vi "Channel Probe_Find Specific VI.vi"(11 "element in":T1) -> (0 "error out":errorcluster, 2 "VI Refnum":refnum<vi>, 3 "element in":T1)   [LabVIEW 2019, in "MessengerM.lvlib"]
uses:
  MessengerM.lvlib
  <vilib>/ChannelSupport/Channel Message/Channel Message.lvclass
  Element.ctl
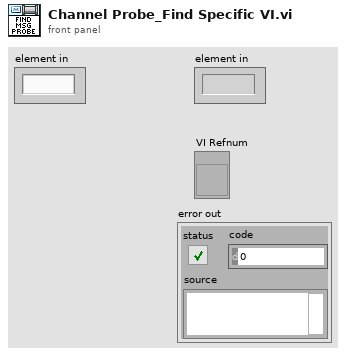
[diagram p1: front panel]
types:
  T1 = typedef "MessengerM.lvlib/Element.ctl" = string
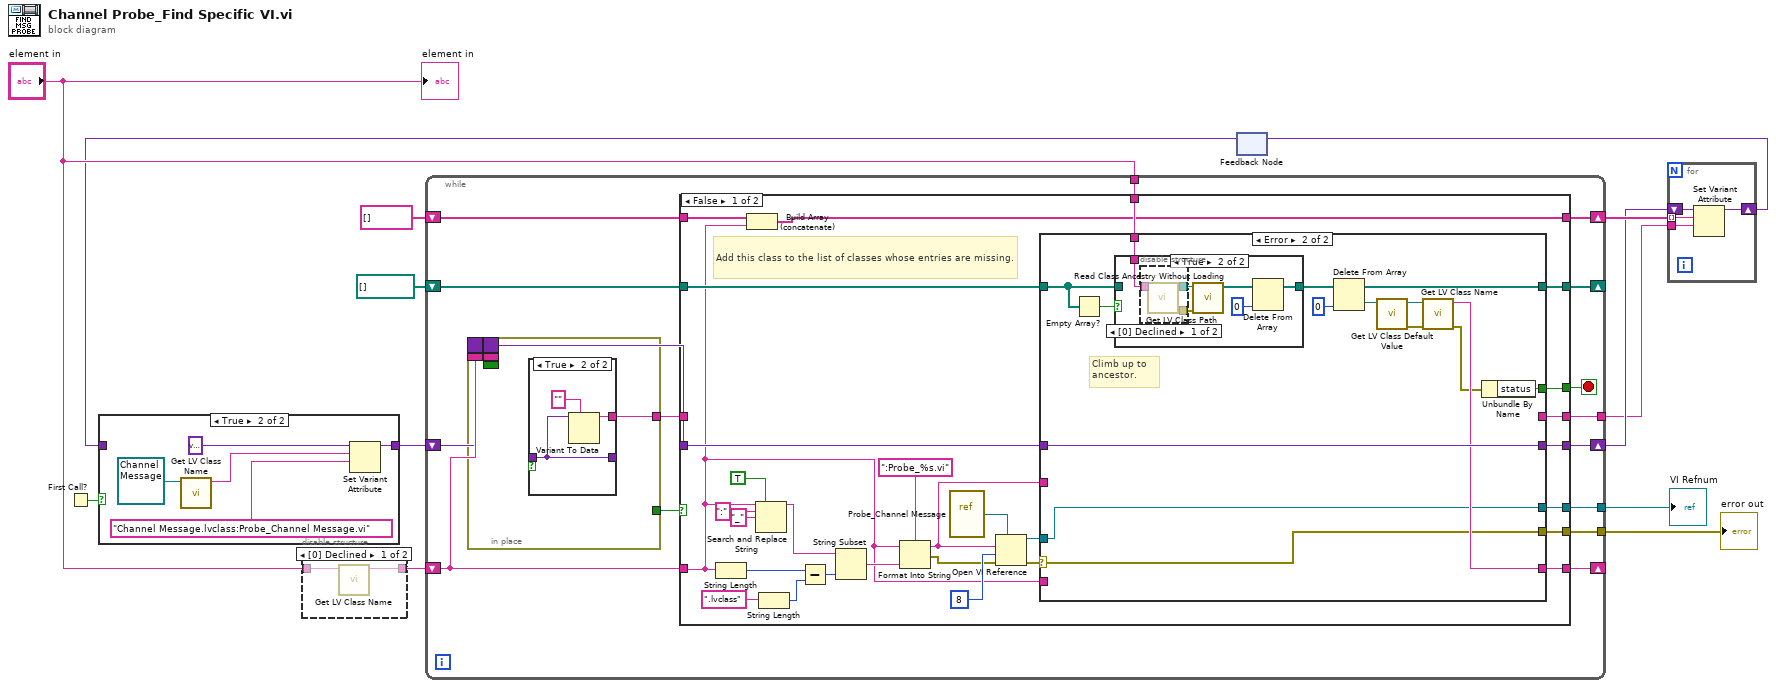
[diagram p0: block diagram]
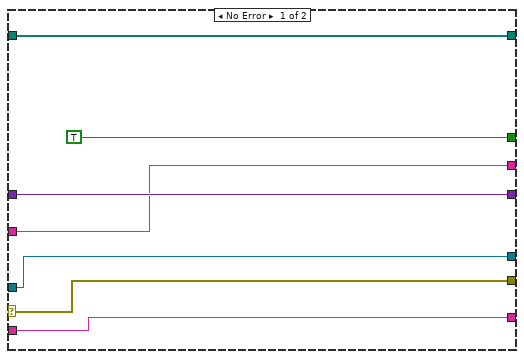
[diagram p4: hidden frame]
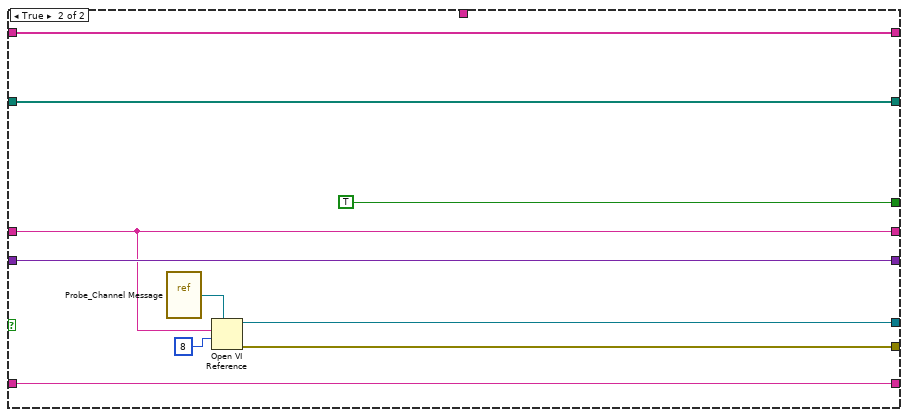
[diagram p7: hidden frame]
diagram:
  n1 = First Call?() -> (First Call?: T/F=w2:bool)
  n2 = disable-structure shown="[0] Declined" {
    disable-tunnel: [w15 _] -> w13
    disable-tunnel: "element in" -> [w14 _]
    frame Disabled {
      n3 = call <vilib>:"Get LV Class Name.vi"("object"=w14) -> ("class name"=w15:string)  [unwired: 9 in, 1 out]
    }
    frame Enabled {
    }
  }
  n4 = feedback #1() -> (w3:variant)  [unwired: 1 in]
  n5 = case shown="True" w2 {
    tunnel: [w16 w19] -> w4
    tunnel: w3 -> [w16 _]
    frame False {
    }
    frame True {
      n6 = call <vilib>:"Get LV Class Name.vi"("object"=refnum<class "Channel Message.lvclass"> refnum ("Channel Message in 2")) -> ("class name"=w18:string)  [unwired: 9 in, 1 out]
      n7 = Set Variant Attribute(Variant=variant, name=w18, value="Channel Message.lvclass:Probe_Channel Message.vi") -> (Variant out=w19:variant)  [unwired: 1 in, 2 out]
    }
  }
  n8 = while {
    shift-right: [w36] -> w6
    shift-left: w4 -> [w23]
    tunnel: [w31] -> w12
    tunnel: [w30] -> w11
    shift-right: [w26] -> _
    shift-left: w13 -> [w32]
    shift-right: [w24] -> w7
    shift-left: string[] [] -> [w25]
    shift-right: [w28] -> _
    shift-left: path[] [] ("Class Ancestry") -> [w29]
    tunnel: "element in" -> [w27]
    tunnel: [w22] -> w1
    stop <- w33 stop-if-true
    n9 = in-place {
      border: w23 -> [_]
      border: w32 -> [_]
      border: [_] -> w35
      border: _ -> [_]
      border: _ -> [_]
      in-place-border: [w39] -> w37
      in-place-border: [w38] -> w34
      n10 = case shown="True" w39 {
        tunnel: [w42 w45] -> w41
        tunnel: w40 -> [w42 w45]
        tunnel: [_ w43] -> w38
        frame False {
        }
        frame True {
          n11 = Variant To Data(type="", Variant=w45) -> (data=w43:string)  [unwired: 1 in, 1 out]
        }
      }
    }
    n12 = case shown="False" w37 {
      tunnel: [w55 w116] -> w36
      tunnel: w35 -> [w63 w116]
      tunnel: [w62 w107] -> w26
      tunnel: w34 -> [_ w108]
      tunnel: [w61 TRUE] -> w33
      tunnel: w32 -> [w47 w107]
      tunnel: [w54 w112] -> w31
      tunnel: [w53 w111] -> w30
      tunnel: w29 -> [w60 w110]
      tunnel: [w59 w110] -> w28
      tunnel: w27 -> [w58 _]
      tunnel: w25 -> [w57 w109]
      tunnel: [w56 w109] -> w24
      tunnel: [w48 w108] -> w22
      frame False {
        # "Add this class to the list of classes whose entries are missing."
        n13 = String Length(string=w47) -> (length=w74:i32)
        n14 = Build Array (concatenate)(w57, w47) -> (w56:string[])
        n15 = Search and Replace String(replace all?=TRUE ("replace all? (F)"), input string=w47, search string=":", replace string="_" ("replace string (\"\")")) -> (result string=w49:string)  [unwired: 4 in, 3 out]
        n16 = String Length(string=".lvclass") -> (length=w72:i32)
        n17 = Subtract(x=w74, y=w72) -> (x-y=w71:i32)
        n18 = String Subset(string=w49, length (rest)=w71) -> (substring=w70:string)  [unwired: 1 in]
        n19 = Format Into String(format string=":Probe_%s.vi", initial string=w47, w70) -> (resulting string=w46:string, error out=w67:errorcluster)  [unwired: 1 in]
        n20 = vi-ref <vilib>:"Probe_Channel Message.vi"() -> (w68:refnum<vi>)
        n21 = Open VI Reference(type specifier VI Refnum (for type only)=w68, vi path=w46, options=8, error in (no error)=w67) -> (vi reference=w65:refnum<vi>, error out=w66:errorcluster)  [unwired: 2 in]
        n22 = case shown="Error" w66 {
          selector: w66 -> [w77 w82]
          tunnel: w65 -> [w78 w83]
          tunnel: w46 -> [w76 _]
          tunnel: w63 -> [w79 w96]
          tunnel: [w75 w86] -> w62
          tunnel: [TRUE w84] -> w61
          tunnel: [w79 w96] -> w55
          tunnel: w60 -> [w80 w94]
          tunnel: [w80 w91] -> w59
          tunnel: w58 -> [_ w93]
          tunnel: [w78 w83] -> w54
          tunnel: [w77 w82] -> w53
          tunnel: [w76 _] -> w48
          tunnel: w47 -> [w75 _]
          frame No Error {
          }
          frame Error {
            # "Climb up to \nancestor."
            n23 = Empty Array?(array=w94) -> (empty?=w95:bool)
            n24 = case shown="True" w95 {
              tunnel: w94 -> [w97 _]
              tunnel: [w97 w99] -> w92
              tunnel: w93 -> [_ w101]
              frame False {
              }
              frame True {
                n25 = disable-structure shown="[0] Declined" {
                  disable-tunnel: [w106 _] -> w103
                  disable-tunnel: [w105 _] -> w102
                  disable-tunnel: w101 -> [w104 _]
                  frame Disabled {
                    n26 = call <vilib>:"Get LV Class Path.vi"("object"=w104) -> ("error out"=w106:errorcluster, "class path"=w105:path)  [unwired: 9 in]
                  }
                  frame Enabled {
                  }
                }
                n27 = call <vilib>:"Read Class Ancestry Without Loading.vi"("error in (no error)"=w103, "LabVIEW Class Path"=w102) -> ("Class Ancestry"=w98:path[])  [unwired: 8 in, 1 out]
                n28 = Delete From Array(array=w98, index=0) -> (array with subset deleted=w99:path[])  [unwired: 1 in, 1 out]
              }
            }
            n29 = Delete From Array(array=w92, index=0) -> (deleted portion=w89:path, array with subset deleted=w91:path[])  [unwired: 1 in]
            n30 = call <vilib>:"Get LV Class Default Value.vi"("class path"=w89) -> ("error out"=w88:errorcluster, "object"=w87:refnum<class>)  [unwired: 9 in]
            n31 = call <vilib>:"Get LV Class Name.vi"("error in (no error)"=w88, "object"=w87) -> ("error out"=w85:errorcluster, "class name"=w86:string)  [unwired: 8 in]
            n32 = Unbundle By Name(w85) -> ("status"=w84:bool)
          }
        }
      }
      frame True {
        n33 = vi-ref <vilib>:"Probe_Channel Message.vi"() -> (w113:refnum<vi>)
        n34 = Open VI Reference(type specifier VI Refnum (for type only)=w113, vi path=w108, options=8) -> (vi reference=w112:refnum<vi>, error out=w111:errorcluster)  [unwired: 3 in]
      }
    }
  }
  "VI Refnum" <- w12
  "error out" <- w11
  n35 = for {
    tunnel: w7 -> [w120] mode=indexing
    tunnel: w1 -> [w118]
    shift-right: [w117] -> w5
    shift-left: w6 -> [w119]
    n36 = Set Variant Attribute(Variant=w119, name=w120, value=w118) -> (Variant out=w117:variant)  [unwired: 1 in, 2 out]
  }
  n37 = feedback-in #1(w5) -> ()
  "element in" <- "element in"
